vi "sub_hasWon.vi"(9 "player":string, 11 "array":string[](array[string])) -> (3 "has won ?":bool)   [LabVIEW 2018]
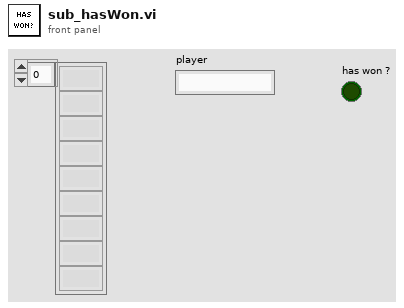
[diagram p1: front panel]
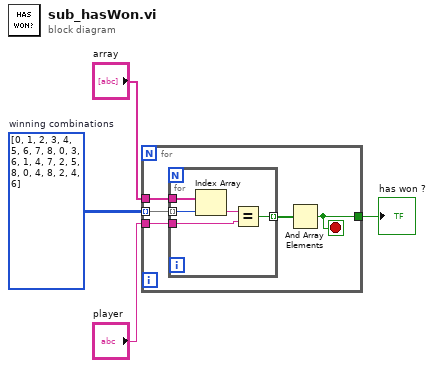
[diagram p0: block diagram]
diagram:
  w3 = i32[][] [[0, 1, 2], [3, 4, 5], [6, 7, 8], [0, 3, 6], [1, 4, 7], [2, 5, 8], [0, 4, 8], [2, 4, 6]]  # winning combinations
  n1 = for {
    tunnel: "array" -> [w9]
    tunnel: w3 -> [w8] mode=indexing
    tunnel: "player" -> [w7]
    tunnel: [w5] -> w1
    stop <- w5 stop-if-true
    n2 = for {
      tunnel: w9 -> [w14]
      tunnel: w8 -> [w13] mode=indexing
      tunnel: w7 -> [w11]
      tunnel: [w10] -> w6 mode=indexing
      n3 = Index Array(array=w14, index=w13) -> (element=w12:string)
      n4 = Equal?(x=w12, y=w11) -> (x = y?=w10:bool)
    }
    n5 = And Array Elements(Boolean array=w6) -> (logical AND=w5:bool)
  }
  "has won ?" <- w1
